vi "Read RP EEPROM Calibration.vi"(8 "error in (no error)":errorcluster, 11 "RP Communicator in":refnum<class "RP Communicator.lvclass">) -> (0 "error out":errorcluster, 2 "RP EEPROM Calibration":T1, 3 "RP Communicator out":refnum<class "RP Communicator.lvclass">)   [LabVIEW 2016, in "RP Communicator.lvclass"]
uses:
  RP Communicator.lvclass
  RP EEPROM Calibration.ctl
  RP Communicator.lvclass/RP Communicator.ctl
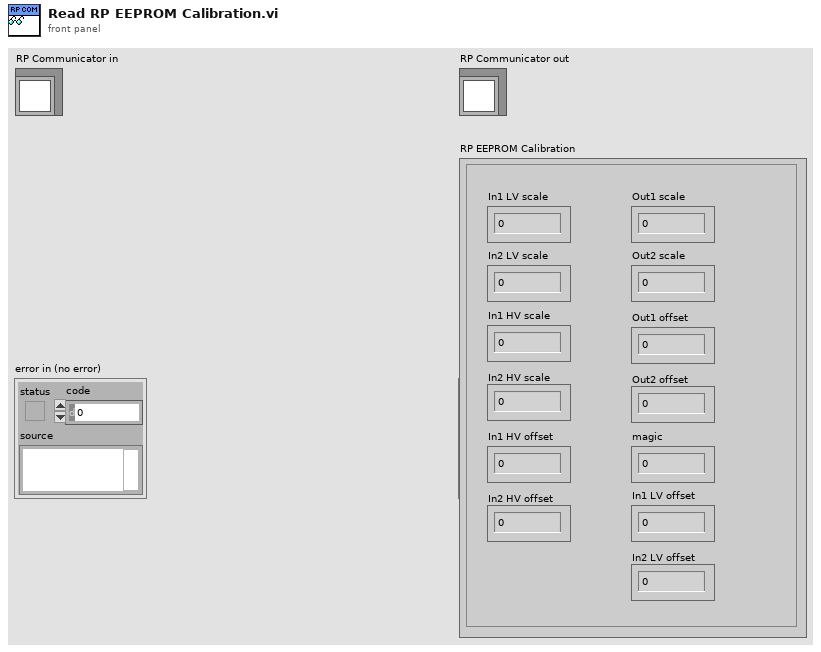
[diagram p1: front panel]
types:
  T1 = typedef "RP EEPROM Calibration.ctl" = cluster{"In1 LV scale":u32, "In2 LV scale":u32, "In1 HV scale":u32, "In2 HV scale":u32, "In1 HV offset":i32, "In2 HV offset":i32, "Out1 scale":u32, "Out2 scale":u32, "Out1 offset":i32, "Out2 offset":i32, "magic":u32, "In1 LV offset":i32, "In2 LV offset":i32}
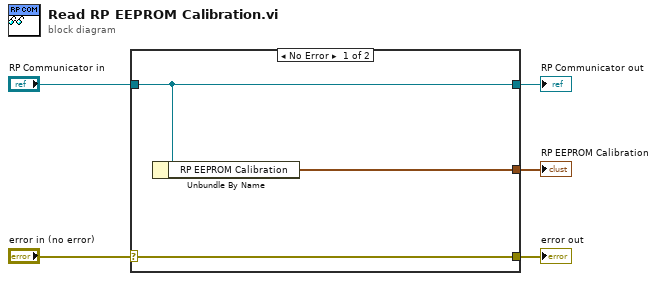
[diagram p0: block diagram]
diagram:
  n1 = case shown="No Error" "error in (no error)" {
    selector: "error in (no error)" -> [w8 w9]
    tunnel: [w8 w9] -> w4
    tunnel: [w7 w10] -> w2
    tunnel: "RP Communicator in" -> [w7 w10]
    tunnel: [w6 _] -> w1
    frame No Error {
      n2 = Unbundle By Name(w7) -> ("RP EEPROM Calibration"=w6:T1)
    }
    frame Error {
    }
  }
  "error out" <- w4
  "RP Communicator out" <- w2
  "RP EEPROM Calibration" <- w1
